vi "TCPIP sender.vi"() -> ()   [LabVIEW 2018]
doc: "Demonstrates how to open a connection to an TCP server, read the data being sent, and display the data on a chart. This VI is designed to stop if the TCP connection is terminated."
uses:
  <vilib>/ErrorRing/Error Ring.xnode
panel:
  in  "Remote TILT":dbl
  in  "Remote PAN":dbl
  in  "Stop":bool
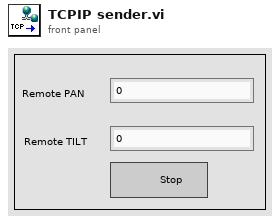
[diagram p1: front panel]
types:
  T1 = enum16{"Init", "Close", "UI events", "Error handler", "Quit"}
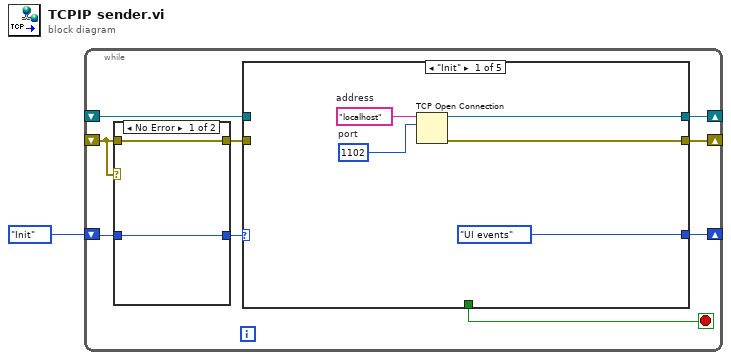
[diagram p0: block diagram]
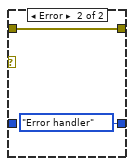
[diagram p2: hidden frame]
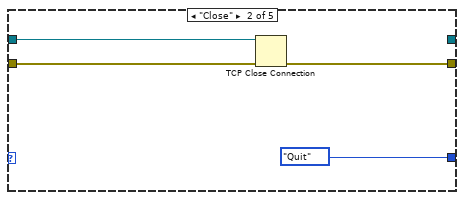
[diagram p3: hidden frame]
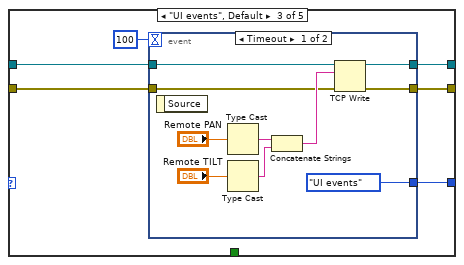
[diagram p4: hidden frame]
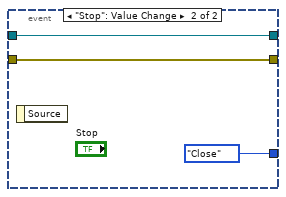
[diagram p5: hidden frame]
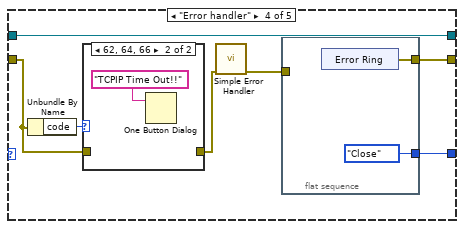
[diagram p6: hidden frame]
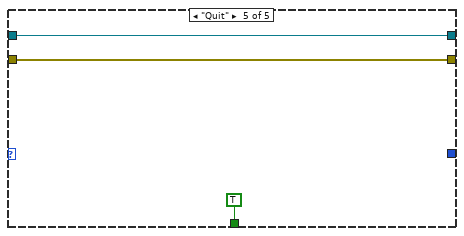
[diagram p8: hidden frame]
diagram:
  n1 = while {
    shift-right: [w8] -> _
    shift-left: T1."Init" -> [w5]
    shift-right: [w10] -> _
    shift-left: _ -> [w9]
    shift-right: [w7] -> _
    shift-left: _ -> [w3]
    stop <- w2 stop-if-true
    n2 = case shown="No Error" w3 {
      tunnel: [w12 T1."Error handler"] -> w6
      tunnel: w5 -> [w12 _]
      tunnel: [w11 w13] -> w4
      tunnel: w3 -> [w11 w13]
      frame No Error {
      }
      frame Error {
      }
    }
    n3 = case shown="\"Init\"" w6 {
      tunnel: [w17 _ w27 w49 w56] -> w10
      tunnel: w9 -> [_ w23 w29 w49 w56]
      tunnel: [T1."UI events" T1."Quit" w26 w47 _] -> w8
      tunnel: [w15 w21 w25 w48 w55] -> w7
      tunnel: w4 -> [_ w22 w24 w44 w55]
      tunnel: [_ _ _ _ TRUE] -> w2
      frame "Init" {
        w18 = u16 1102  # port
        w19 = "localhost"  # address
        n4 = TCP Open Connection(address=w19, remote port or service name=w18) -> (connection ID=w17:refnum<k5>, error out=w15:errorcluster)  [unwired: 3 in]
      }
      frame "Close" {
        n5 = TCP Close Connection(connection ID=w23, error in (no error)=w22) -> (error out=w21:errorcluster)  [unwired: 1 in, 1 out]
      }
      frame "UI events", Default {
        n6 = event shown="[0] Timeout" {
          selector: _ -> [_ _]
          dyn-events: _ -> [_ _]
          timeout: 100 -> [_ _]
          tunnel: w29 -> [w35 w40]
          tunnel: [w34 w40] -> w27
          tunnel: [T1."UI events" T1."Close"] -> w26
          tunnel: [w31 w41] -> w25
          tunnel: w24 -> [w30 w41]
          event Timeout {
            n7 = event-data() -> ()  [unwired: 1 in, 1 out]
            n8 = Type Cast(x="Remote PAN") -> (*(type *) &x=w38:string)  [unwired: 1 in]
            n9 = Type Cast(x="Remote TILT") -> (*(type *) &x=w39:string)  [unwired: 1 in]
            n10 = Concatenate Strings(w38, w39) -> (w33:string)
            n11 = TCP Write(connection ID=w35, data in=w33, error in (no error)=w30) -> (connection ID out=w34:refnum<k5>, error out=w31:errorcluster)  [unwired: 2 out]
          }
          event "Stop": Value Change {
            n12 = event-data() -> ()  [unwired: 1 in, 1 out]
          }
        }
      }
      frame "Error handler" {
        n13 = Unbundle By Name(w44) -> ("code"=w45:i32)
        n14 = case shown="62, 64, 66" w45 {
          tunnel: w44 -> [w50 _]
          tunnel: [w50 _] -> w43
          frame Default {
          }
          frame 62, 64, 66 {
            n15 = One Button Dialog(message="TCPIP Time Out!!") -> ()  [unwired: 1 in, 1 out]
          }
        }
        n16 = call <vilib>:"Simple Error Handler.vi"("error in (no error)"=w43) -> ("error out"=w46:errorcluster)  [unwired: 4 in, 4 out]
        n17 = flat-sequence {
          tunnel: [w53] -> w48
          tunnel: [T1."Close"] -> w47
          tunnel: w46 -> [_]
          frame #0 {
            n18 = xnode "Error Ring"() -> ("error out"=w53:errorcluster)
          }
        }
      }
      frame "Quit" {
      }
    }
  }
